vi "Facade.vi"(0 "Data In":T5, 2 "Display State In":T3, 3 "Container State":T4) -> (6 "Data Out":T5, 7 "Display State Out":T3, 8 "Action":T2)   [LabVIEW 2021, in "myRIO MSP.xctl"]
uses:
  <vilib>/myRIO/Common/Instrument Driver Framework/Utilities/xctls/myRIO MSP/myRIO MSP.xctl
  <vilib>/myRIO/Common/Instrument Driver Framework/Utilities/xctls/myRIO MSP/Data.ctl
  <vilib>/_xctls/Container State.ctl
  <vilib>/myRIO/Common/Instrument Driver Framework/Utilities/xctls/myRIO MSP/State.ctl
  <vilib>/_xctls/Action.ctl
  <vilib>/_xctls/XControlSupport.lvlib
panel:
  in  "MSP":T1
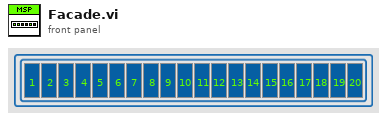
[diagram p1: front panel]
types:
  T1 = cluster{"1":bool, "2":bool, "3":bool, "4":bool, "5":bool, "6":bool, "7":bool, "8":bool, "9":bool, "10":bool, "11":bool, "12":bool, "13":bool, "14":bool, "15":bool, "16":bool, "17":bool, "18":bool, "19":bool, "20":bool}
  T2 = typedef "XControlSupport.lvlib/Action.ctl" = cluster{"Data Changed?":bool, "State Changed?":bool, "Action Name":string}
  T3 = typedef "myRIO MSP.xctl/State.ctl" = cluster{"Pin Disabled?":enum8{"Enabled", "Disabled", "Disabled and Grayed Out"}[], "Pin Name":string[]}
  T4 = typedef "XControlSupport.lvlib/Container State.ctl" = cluster{"Indicator?":bool, "Run Mode?":bool, " Refnum":refnum<vi>}
  T5 = typedef "myRIO MSP.xctl/Data.ctl" = bool[]
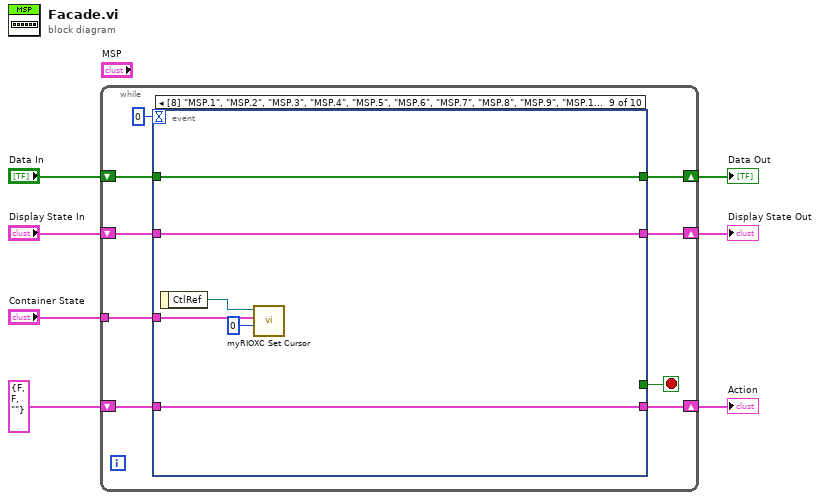
[diagram p0: block diagram]
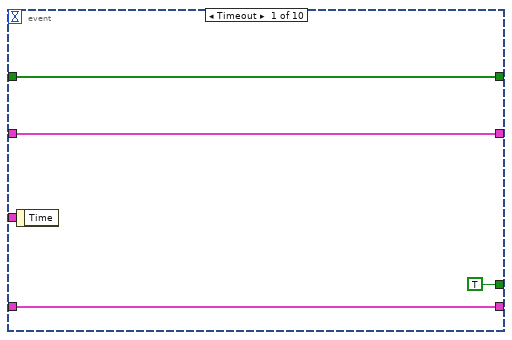
[diagram p2: hidden frame]
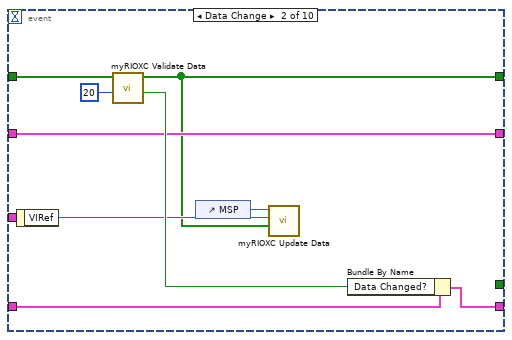
[diagram p3: hidden frame]
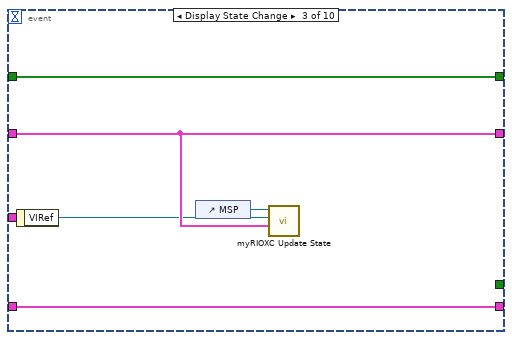
[diagram p4: hidden frame]
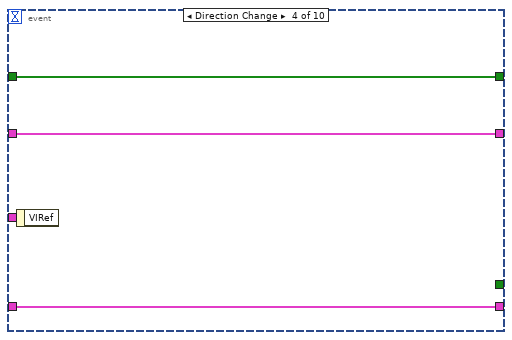
[diagram p5: hidden frame]
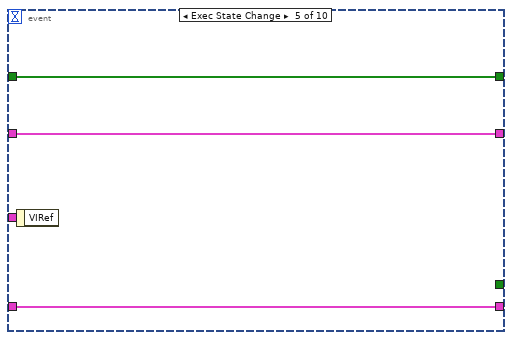
[diagram p6: hidden frame]
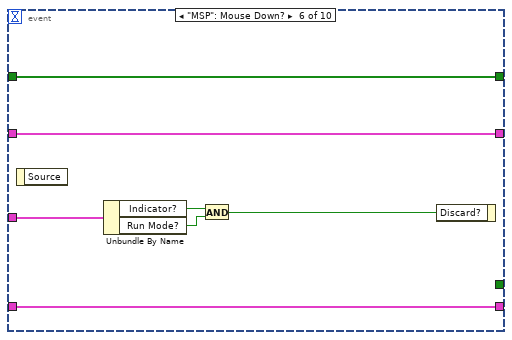
[diagram p7: hidden frame]
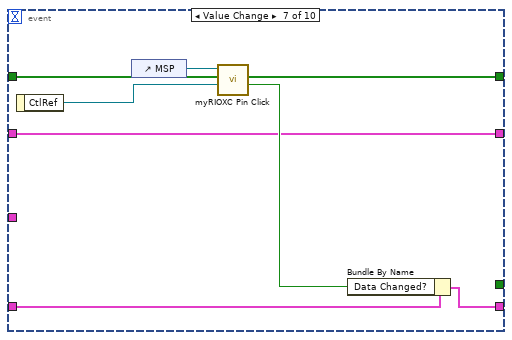
[diagram p8: hidden frame]
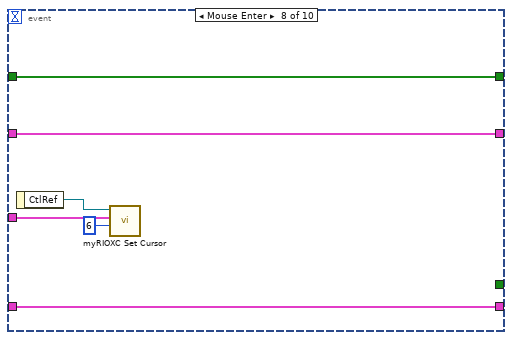
[diagram p9: hidden frame]
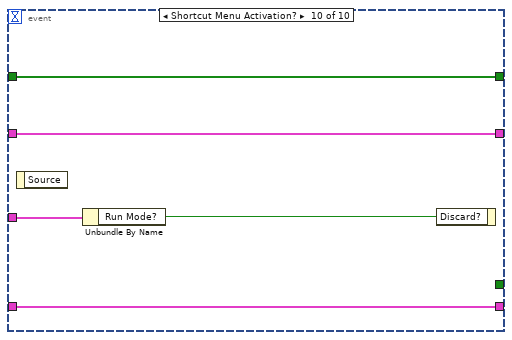
[diagram p10: hidden frame]
diagram:
  n1 = while {
    shift-right: [w16] -> w4
    shift-left: "Display State In" -> [w8]
    tunnel: "Container State" -> [w10]
    shift-right: [w13] -> w7
    shift-left: "Data In" -> [w11]
    shift-right: [w12] -> w2
    shift-left: T2 {"Data Changed?"=FALSE, "State Changed?"=FALSE, "Action Name"=""} ("Action") -> [w9]
    stop <- w15 stop-if-true
    n2 = event shown="[8] \"MSP.1\", \"MSP.2\", \"MSP.3\", \"MSP.4\", \"MSP.5\", \"MSP.6\", \"MSP.7\", \"MSP.8\", \"MSP.9\", \"MSP.10\", \"MSP.11\", \"MSP.12\", \"MSP.13\", \"MSP.14\", \"MSP.15\", \"MSP.16\", \"MSP.17\", \"MSP.18\", \"MSP.19\", \"MSP.20\": Mouse Leave" {
      selector: _ -> [_ _ _ _ _ _ _ _ _ _]
      dyn-events: _ -> [_ _ _ _ _ _ _ _ _ _]
      timeout: 0 -> [_ _ _ _ _ _ _ _ _ _]
      tunnel: w8 -> [w18 w24 w33 w35 w39 w47 w54 w61 w67 w72]
      tunnel: [w18 w24 w33 w35 w39 w47 w54 w61 w67 w72] -> w16
      tunnel: [TRUE _ _ _ _ _ _ _ _ _] -> w15
      tunnel: w10 -> [_ _ _ _ _ w41 _ w56 w63 w69]
      tunnel: w11 -> [w17 w29 w34 w37 w40 w46 w49 w60 w66 w71]
      tunnel: [w17 w21 w34 w37 w40 w46 w48 w60 w66 w71] -> w13
      tunnel: [w19 w26 w32 w36 w38 w45 w52 w59 w65 w70] -> w12
      tunnel: w9 -> [w19 w27 w32 w36 w38 w45 w53 w59 w65 w70]
      event Timeout {
        n3 = event-data() -> ()  [unwired: 1 in, 1 out]
      }
      event Data Change {
        n4 = event-data() -> ("VIRef"=w22:refnum<vi>)  [unwired: 1 in]
        n5 = call <vilib>:"myRIOXC Validate Data.vi"("Size"=20, "Data In"=w29) -> ("Data Changed?"=w25:bool, "Data Out"=w21:bool[])  [unwired: 8 in]
        n6 = control-ref of="MSP"() -> (w23:refnum<vi>)
        n7 = call <vilib>:"myRIOXC Update Data.vi"("Data In"=w21, "Facade Ref"=w22, "Connector Ref"=w23) -> ()  [unwired: 8 in, 1 out]
        n8 = Bundle By Name(cluster=w27, "Data Changed?"=w25) -> (w26:T2)
      }
      event Display State Change {
        n9 = event-data() -> ("VIRef"=w30:refnum<vi>)  [unwired: 1 in]
        n10 = control-ref of="MSP"() -> (w31:refnum<vi>)
        n11 = call <vilib>:"myRIOXC Update State.vi"("Display State In"=w33, "Facade Ref"=w30, "Connector Ref"=w31) -> ()  [unwired: 8 in, 1 out]
      }
      event Direction Change {
        n12 = event-data() -> ()  [unwired: 1 in, 1 out]
      }
      event Exec State Change {
        n13 = event-data() -> ()  [unwired: 1 in, 1 out]
      }
      event "MSP": Mouse Down? {
        n14 = event-data() -> ()  [unwired: 1 in, 1 out]
        n15 = Unbundle By Name(w41) -> ("Indicator?"=w44:bool, "Run Mode?"=w43:bool)
        n16 = And(x=w44, y=w43) -> (x .and. y?=w42:bool)
        n17 = event-data("Discard?"=w42) -> ()  [unwired: 1 in, 1 out]
      }
      event "MSP.1", "MSP.2", "MSP.3", "MSP.4", "MSP.5", "MSP.6", "MSP.7", "MSP.8", "MSP.9", "MSP.10", "MSP.11", "MSP.12", "MSP.13", "MSP.14", "MSP.15", "MSP.16", "MSP.17", "MSP.18", "MSP.19", "MSP.20": Value Change {
        # "Value Change"
        n18 = event-data() -> ("CtlRef"=w51:refnum<vi>)  [unwired: 1 in]
        n19 = control-ref of="MSP"() -> (w50:refnum<vi>)
        n20 = call <vilib>:"myRIOXC Pin Click.vi"("Pin Ref"=w51, "Data In"=w49, "Connector Ref"=w50) -> ("Value Change?"=w55:bool, "Data Out"=w48:bool[])  [unwired: 6 in, 1 out]
        n21 = Bundle By Name(cluster=w53, "Data Changed?"=w55) -> (w52:T2)
      }
      event "MSP.1", "MSP.2", "MSP.3", "MSP.4", "MSP.5", "MSP.6", "MSP.7", "MSP.8", "MSP.9", "MSP.10", "MSP.11", "MSP.12", "MSP.13", "MSP.14", "MSP.15", "MSP.16", "MSP.17", "MSP.18", "MSP.19", "MSP.20": Mouse Enter {
        n22 = event-data() -> ("CtlRef"=w57:refnum<vi>)  [unwired: 1 in]
        n23 = call <vilib>:"myRIOXC Set Cursor.vi"("Cursor"=u16 6, "Container State"=w56, "PIN Ref"=w57) -> ()  [unwired: 9 in]
      }
      event "MSP.1", "MSP.2", "MSP.3", "MSP.4", "MSP.5", "MSP.6", "MSP.7", "MSP.8", "MSP.9", "MSP.10", "MSP.11", "MSP.12", "MSP.13", "MSP.14", "MSP.15", "MSP.16", "MSP.17", "MSP.18", "MSP.19", "MSP.20": Mouse Leave {
        n24 = event-data() -> ("CtlRef"=w62:refnum<vi>)  [unwired: 1 in]
        n25 = call <vilib>:"myRIOXC Set Cursor.vi"("Cursor"=u16 0, "Container State"=w63, "PIN Ref"=w62) -> ()  [unwired: 9 in]
      }
      event Shortcut Menu Activation? {
        n26 = event-data() -> ()  [unwired: 1 in, 1 out]
        n27 = Unbundle By Name(w69) -> ("Run Mode?"=w68:bool)
        n28 = event-data("Discard?"=w68) -> ()  [unwired: 1 in, 1 out]
      }
    }
  }
  "Display State Out" <- w4
  "Data Out" <- w7
  "Action" <- w2
